vi "EMD8216 WDT set.vi"(9 "state":u8[](array[numeric]), 10 "time":u16, 11 "CardID":u32) -> (3 "error_code":u32)   [LabVIEW 2009, in "EMD8216_64.lvlib"]
doc: "EMD8216Status EMD8216_WDT_set(u32 CardID,u16 time,u8 state[2]);"
uses:
  EMD8216_64.lvlib
  <userlib>/EMD8216_64/EMD8216_64.dll
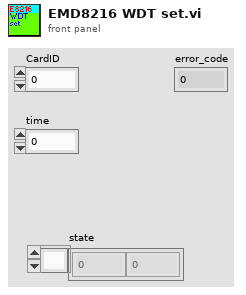
[diagram p1: front panel]
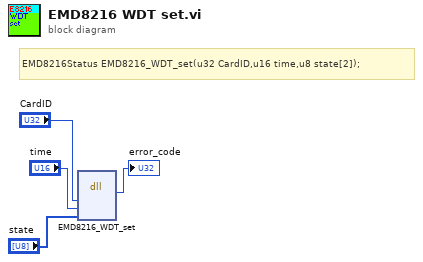
[diagram p0: block diagram]
diagram:
  # "EMD8216Status EMD8216_WDT_set(u32 CardID,u16 time,u8 state[2]);"
  n1 = dll-call lib="C:/Program Files/National Instruments/LabVIEW 2017/user.lib/EMD8216_64/EMD8216_64.*" fn="EMD8216_WDT_set"("CardID"="CardID", "time"="time", "state"="state") -> ("return type"=→"error_code":u32)  [unwired: 6 in, 2 out]
